vi "RSZVL_GetFreqOfPeakPower.vi"(0 "VISA resource name":refnum<visa-resource-name>, 1 "Center Freq.":dbl caption="Center Freq. (Hz)", 2 "Freq. Span":dbl caption="Freq. Span (Hz)", 3 "Expected Power":dbl caption="Expected Power (dBm)", 4 "Ref. Level":dbl caption="Ref. Level (dBm)", 5 "error in (no error)":errorcluster {"code" format="%.0x"}, 7 "Calibration Enabled":bool, 8 "Auto Center":bool=TRUE, 9 "Route Names":string[](array[string])) -> (10 "Found":bool, 14 "Marker Freq.":dbl, 16 "Marker Power Calibrated":dbl=-9.89595207905 caption="Measured Power Calibrated", 17 "Marker Power Raw":dbl=-9.89595207905, 19 "error out":errorcluster {"code" format="%.0x"})   [LabVIEW 2015]
doc: "This Vi is used to find the Frequency of peak power, using R&S ZVL Spectrum Analyzer. \nThis Vi can be used to validate peak power is at the expected frequency.\n\n1- Spec. An is placed at Center freq. with specified Span (span should be just wide enough to catch the peak power)- Peak Power and its frequency are measured\n\n2- If Auto Center option is selected, the Spec An is re-centered after the intial found peak power, and Span is set to 1MHZ for better resolution and accuracy and Peak Power frequency is measured again.\n\nSearched Peak Power must be within 85% of specified Expected Power to be considered found. Will make number of attempts (for pulsed power) to find the Peak Power."
panel:
  # "Get Peak Power Frequency"
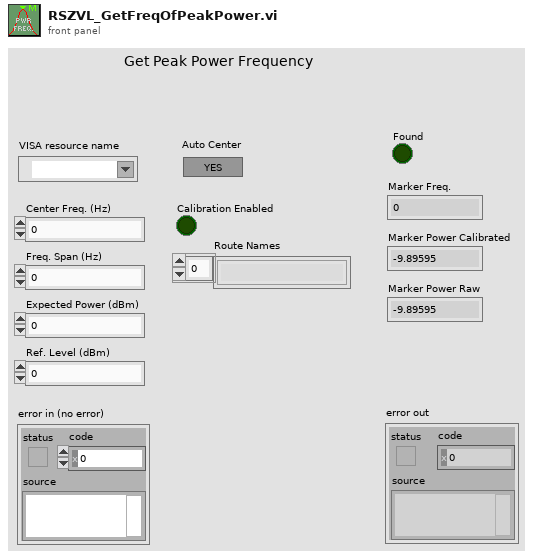
[diagram p1: front panel]
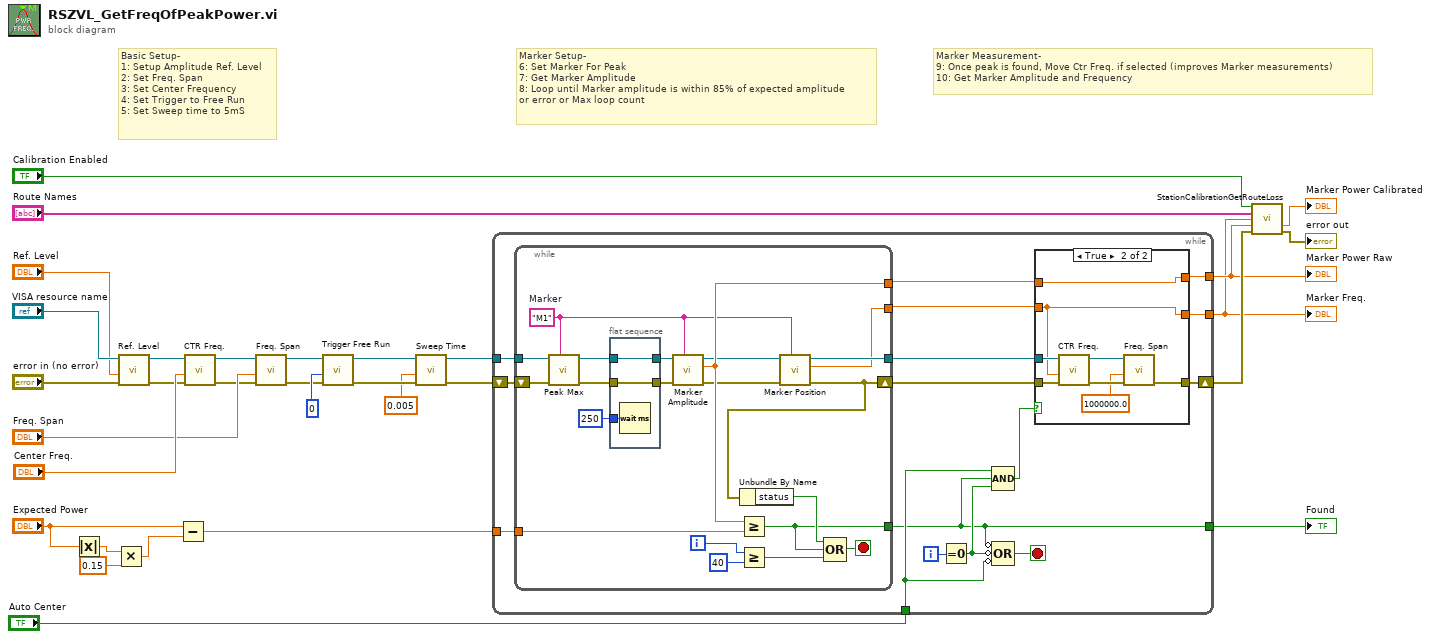
[diagram p0: block diagram]
diagram:
  # "Marker Measurement-\n9: Once peak is found, Move Ctr Freq. if selected (improves Marker measurements)\n10: Get Marker Amplitude and Frequency"
  # "Marker Setup-\n6: Set Marker For Peak\n7: Get Marker Amplitude\n8: Loop until Marker amplitude is within 85% of expected amplitude\nor error or Max loop count"
  # "Basic Setup-\n1: Setup Amplitude Ref. Level\n2: Set Freq. Span\n3: Set Center Frequency\n4: Set Trigger to Free Run\n5: Set Sweep time to 5mS"
  n1 = Absolute Value(x="Expected Power") -> (abs(x)=w26:dbl)
  n2 = Multiply(x=w26, y=0.15) -> (x*y=w23:dbl)
  n3 = call "Ref. Level"("error in (no error)"="error in (no error)", "Input Double"="Ref. Level", "instrument handle"="VISA resource name") -> ("error out"=w18:errorcluster, "instrument handle out"=w19:refnum<visa-resource-name>)  [unwired: 7 in]
  n4 = Subtract(x="Expected Power", y=w23) -> (x-y=w22:dbl)
  n5 = call "CTR Freq."("error in (no error)"=w18, "Input Double"="Center Freq.", "instrument handle"=w19) -> ("error out"=w16:errorcluster, "instrument handle out"=w17:refnum<visa-resource-name>)  [unwired: 7 in]
  n6 = call "Freq. Span"("error in (no error)"=w16, "Input Double"="Freq. Span", "instrument handle"=w17) -> ("error out"=w13:errorcluster, "instrument handle out"=w14:refnum<visa-resource-name>)  [unwired: 7 in]
  n7 = call "Trigger Free Run"("error in (no error)"=w13, "Input I32"=0, "instrument handle"=w14) -> ("error out"=w11:errorcluster, "instrument handle out"=w12:refnum<visa-resource-name>)  [unwired: 7 in]
  n8 = call "Sweep Time"("error in (no error)"=w11, "Input Double"=0.005, "instrument handle"=w12) -> ("error out"=w9:errorcluster, "instrument handle out"=w10:refnum<visa-resource-name>)  [unwired: 7 in]
  n9 = while {
    tunnel: w10 -> [w47]
    tunnel: w22 -> [w45]
    tunnel: [w42] -> w5
    tunnel: [w41] -> w6
    tunnel: [w32] -> w21
    tunnel: "Auto Center" -> [w33]
    shift-right: [w40] -> w7
    shift-left: w9 -> [w46]
    i -> [w36]
    stop <- w35 stop-if-true
    n10 = while {
      tunnel: w47 -> [w78]
      shift-right: [w61] -> w43
      shift-left: w46 -> [w76]
      tunnel: w45 -> [w74]
      tunnel: [w68] -> w32
      tunnel: [w62] -> w44
      tunnel: [w65] -> w39
      tunnel: [w60] -> w38
      i -> [w73]
      stop <- w69 stop-if-true
      w59 = "M1"  # Marker
      n11 = call "Peak Max"("Repeated Capabilities"=w59, "error in (no error)"=w76, "instrument handle"=w78) -> ("error out"=w75:errorcluster, "instrument handle out"=w77:refnum<visa-resource-name>)  [unwired: 7 in]
      n12 = flat-sequence {
        tunnel: w77 -> [w82]
        tunnel: [w82] -> w67
        tunnel: w75 -> [w81]
        tunnel: [w81] -> w66
        tunnel: u32 250 ("Input I32") -> [w80]
        frame #0 {
          n13 = Wait (ms)(milliseconds to wait=w80) -> ()  [unwired: 1 out]
        }
      }
      n14 = call "Marker Amplitude"("Repeated Capabilities"=w59, "error in (no error)"=w66, "instrument handle"=w67) -> ("error out"=w63:errorcluster, "Output Double"=w65:dbl, "instrument handle out"=w64:refnum<visa-resource-name>)  [unwired: 6 in]
      n15 = Greater Or Equal?(x=w65, y=w74) -> (x >= y?=w68:bool)
      n16 = Greater Or Equal?(x=w73, y=40) -> (x >= y?=w70:bool)
      n17 = call "Marker Position"("Repeated Capabilities"=w59, "error in (no error)"=w63, "instrument handle"=w64) -> ("error out"=w61:errorcluster, "Output Double"=w60:dbl, "instrument handle out"=w62:refnum<visa-resource-name>)  [unwired: 6 in]
      n18 = Unbundle By Name(w61) -> ("status"=w71:bool)
      n19 = Compound Arithmetic op=OR(w71, w68, w70) -> (w69:bool)
    }
    n20 = Equal To 0?(x=w36) -> (x = 0?=w34:bool)
    n21 = Compound Arithmetic op=AND(w33, w32, w34) -> (w37:bool)
    n22 = Compound Arithmetic op=OR(invert w32, invert w34, invert w33) -> (w35:bool)
    n23 = case shown="True" w37 {
      tunnel: w44 -> [_ w58]
      tunnel: w43 -> [w49 w57]
      tunnel: [w48 w55] -> w42
      tunnel: [w50 w56] -> w41
      tunnel: [w49 w52] -> w40
      tunnel: w39 -> [w50 w56]
      tunnel: w38 -> [w48 w55]
      frame False {
      }
      frame True {
        n24 = call "CTR Freq."("error in (no error)"=w57, "Input Double"=w55, "instrument handle"=w58) -> ("error out"=w54:errorcluster, "instrument handle out"=w53:refnum<visa-resource-name>)  [unwired: 7 in]
        n25 = call "Freq. Span"("error in (no error)"=w54, "Input Double"=1000000.0, "instrument handle"=w53) -> ("error out"=w52:errorcluster)  [unwired: 7 in, 1 out]
      }
    }
  }
  "Marker Freq." <- w5
  "Marker Power Raw" <- w6
  "Found" <- w21
  n26 = call "StationCalibrationGetRouteLoss.vi"("Calibration Enabled"="Calibration Enabled", "Route Names"="Route Names", "Frequency"=w5, "Power Level"=w6, "error in (no error)"=w7) -> ("Adjusted Power Level"=→"Marker Power Calibrated":dbl, "error out"=→"error out":errorcluster)  [unwired: 7 in, 2 out]
